vi "sample5(Wrapper).vi"() -> ()   [LabVIEW 2011]
uses:
  <vilib>/Platform/TimedLoop/XDataNode/timing_clust.ctl
  <vilib>/Platform/TimedLoop/XDataNode/nitl_modes.ctl
  <vilib>/Platform/TimedLoop/XDataNode/wakeup.ctl
  <vilib>/Platform/TimedLoop/XDataNode/XDataNode.xnode
  <vilib>/Platform/TimedLoop/XDataNode/XDNodeRunTimeDep.lvlib
panel:
  in  "OffsetTime":u32=20
  out "Present Speed":i16
  in  "waveform":enum16{"sin", "square"}(ring)
  in  "freq":dbl=0.3 format="%_3f"
  in  "Acceleration":u8 max=254
  in  "Goal Speed":i16 min=-1023 max=1023
  out "CycleTime2":dbl format="%.2g"
  out "Load":i16
  in  "TorqueLimit":u16 max=1023
  in  "PID_Gain":u8[](array[numeric])=[0, 0, 0] max=254
  in  "Target ID":u8=1 max=253
  in  "Baudrate":u32=1000000 min=8000 max=3000000
  in  "COM":refnum<visa-resource-name> caption="COMポート"
  out "CycleTime1":dbl format="%.2g"
  out "Current":i16
  in  "wave":bool
  out "CtrlTable":u8[](array[numeric]) format="%02x"
  out "Chart":T1(graph)
  out "STOP2":bool
  out "Present Pos":u16
  in  "STOP":bool
  in  "Goal Pos":u16(knob) scale=0.0..4095.0
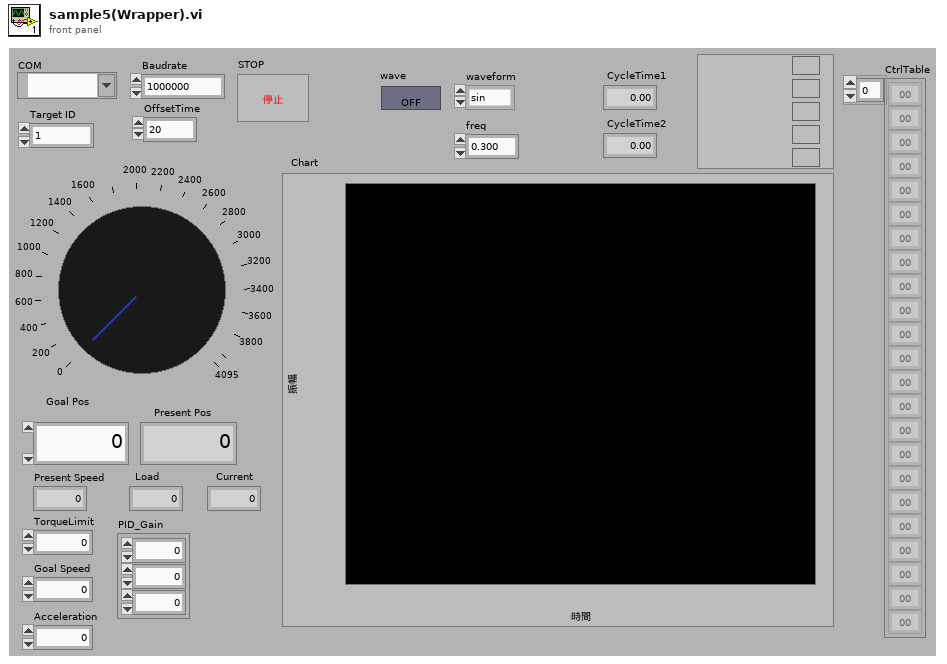
[diagram p1: front panel]
types:
  T1 = cluster{"Goal Pos":u16, "Present Pos":u16, "Current":i16, "Load":i16, "Present Speed":i16}
  T2 = typedef "XDNodeRunTimeDep.lvlib/timing_clust.ctl" = cluster{"Expected End [f-1]":u64, "Actual End [f-1]":u64, "Finished Late? [f-1]":bool, "Expected End [i-1]":u64, "Actual End [i-1]":u64, "Finished Late? [i-1]":bool, "Expected Start [i]":u64, "Actual Start [i]":u64, "Expected Start [f]":u64, "Actual Start [f]":u64, "Source Name":string, "Structure Name":string, "Period":i64, "Deadline":i64, "Offset":i64, "Start":i64, "Priority":i32, "Timeout":i32, "Mode":T3, "Wakeup Reason":T4, "Error":errorcluster, "Source Type":string, "Secondary Source Type":string, "Global End Time":u64, "Global Start Time":u64, "Frame Duration":u64, "Iteration Duration":u64, "Assigned CPU":i32, "I/O Scan Engine Mode":u32}
  T3 = typedef "XDNodeRunTimeDep.lvlib/nitl_modes.ctl" = enum32{"No Change", "Process missed periods, maintain original phase", "Discard missed periods, maintain original phase", "Process missed periods, ignore original phase", "Discard missed periods, ignore original phase"}
  T4 = typedef "XDNodeRunTimeDep.lvlib/wakeup.ctl" = enum32{"Normal", "Aborted", "Asynchronous wakeup", "Timing source error", "Timed loop error", "Timeout"}
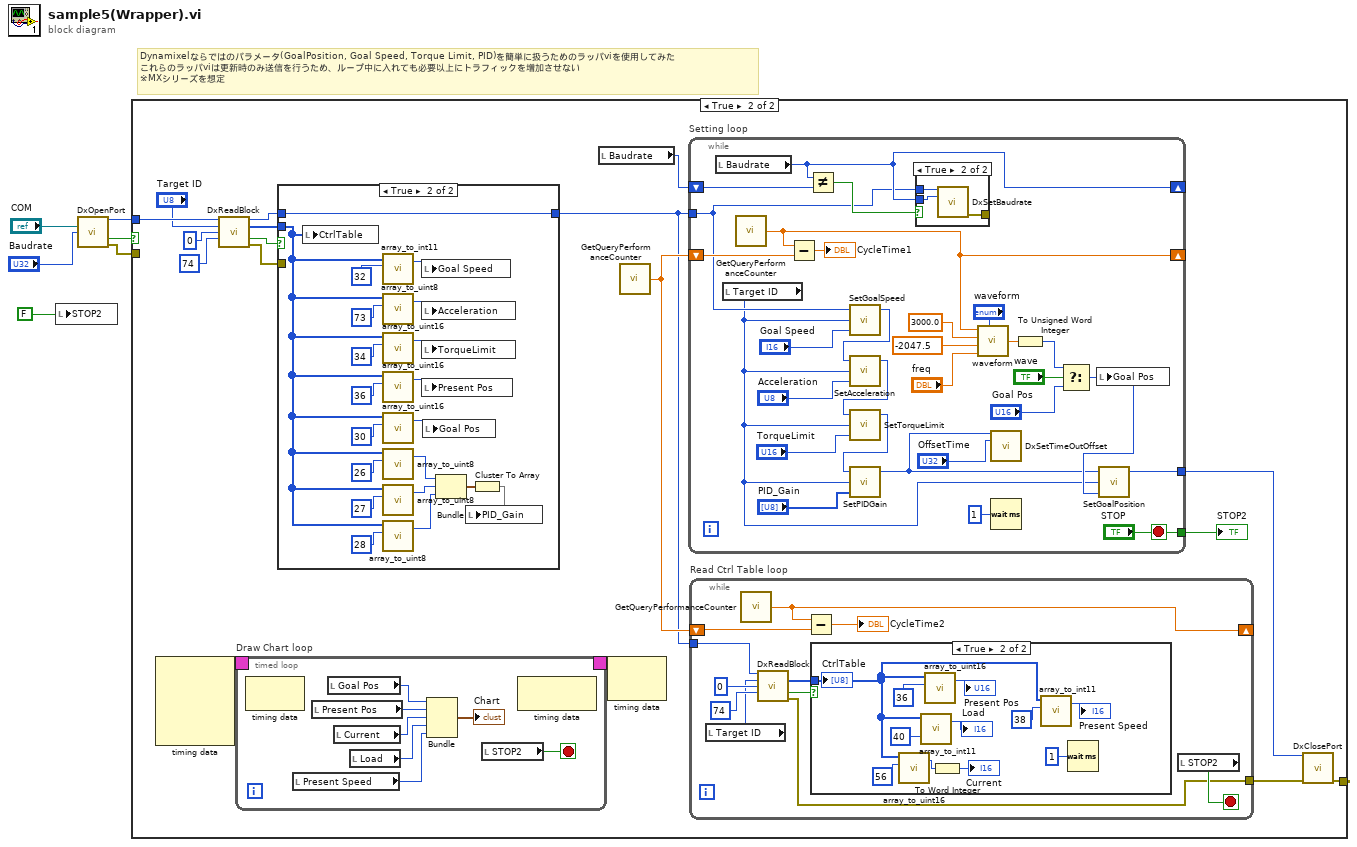
[diagram p0: block diagram]
diagram:
  # "Dynamixelならではのパラメータ(GoalPosition, Goal Speed, Torque Limit, PID)を簡単に扱うためのラッパviを使用してみた\nこれらのラッパviは更新時のみ送信を行うため、ループ中に入れても必要以上にトラフィックを増加させない\n※MXシリーズを想定"
  n1 = local write "STOP2"(FALSE ("停止 3")) -> ()
  n2 = call "DxOpenPort.vi"("port"="COM", "baudrate"="Baudrate") -> ("dvid"=w5:u32, "成功"=w4:bool, "エラー出力"=w6:errorcluster)  [unwired: 11 in]
  n3 = case shown="TRUE" w4 {
    tunnel: w6 -> [_ _]
    tunnel: w5 -> [_ w16]
    tunnel: [_ w9] -> _
    frame False {
    }
    frame True {
      n4 = node-c288() -> (w22:T2)  [unwired: 4 in]
      n5 = call "DxReadBlock.vi"("dvid in"=w16, "id"="Target ID", "address"=u16 0 ("pos"), "size"=u32 74) -> ("dvid out"=w12:u32, "data out"=w14:u8[], "成功"=w13:bool, "エラー出力"=w10:errorcluster)  [unwired: 8 in]
      n6 = timed-loop "Draw Chart loop" {
        timing: w22 -> [_]
        timing-out: [_] -> w21
        stop <- w51 stop-if-true
        n7 = node-c288() -> ()  [unwired: 1 in, 1 out]
        n8 = local read "Present Speed"() -> (w45:i16)
        n9 = local read "Present Pos"() -> (w49:u16)
        n10 = local read "Goal Pos"() -> (w50:u16)
        n11 = local read "Current"() -> (w47:i16)
        n12 = local read "Load"() -> (w46:i16)
        n13 = Bundle("Goal Pos"=w50, "Present Pos"=w49, "Current"=w47, "Load"=w46, "Present Speed"=w45) -> (→"Chart":T1)  [unwired: 1 in]
        n14 = local read "STOP2"() -> (w51:bool)
        n15 = node-c288() -> ()  [unwired: 1 in, 1 out]
      }
      n16 = case shown="TRUE" w13 {
        tunnel: w14 -> [_ w26]
        tunnel: w12 -> [w24 w28]
        tunnel: [w24 w28] -> w11
        tunnel: w10 -> [_ _]
        frame False {
        }
        frame True {
          n17 = local write "CtrlTable"(w26) -> ()
          n18 = call "array_to_int11.vi"("OffsetAddr"=u16 32, "array"=w26) -> ("int16"=w25:i16)  [unwired: 5 in]
          n19 = call "array_to_uint8.vi"("OffsetAddr"=u16 73, "array"=w26) -> ("uint8"=w43:u8)  [unwired: 5 in]
          n20 = call "array_to_uint16.vi"("OffsetAddr"=u16 34, "array"=w26) -> ("uint16"=w37:u16)  [unwired: 5 in]
          n21 = call "array_to_uint16.vi"("OffsetAddr"=u16 36, "array"=w26) -> ("uint16"=w41:u16)  [unwired: 5 in]
          n22 = call "array_to_uint16.vi"("OffsetAddr"=u16 30, "array"=w26) -> ("uint16"=w40:u16)  [unwired: 5 in]
          n23 = call "array_to_uint8.vi"("OffsetAddr"=u16 26, "array"=w26) -> ("uint8"=w33:u8)  [unwired: 5 in]
          n24 = call "array_to_uint8.vi"("OffsetAddr"=u16 27, "array"=w26) -> ("uint8"=w32:u8)  [unwired: 5 in]
          n25 = call "array_to_uint8.vi"("OffsetAddr"=u16 28, "array"=w26) -> ("uint8"=w31:u8)  [unwired: 5 in]
          n26 = local write "Goal Speed"(w25) -> ()
          n27 = local write "Acceleration"(w43) -> ()
          n28 = local write "TorqueLimit"(w37) -> ()
          n29 = local write "Present Pos"(w41) -> ()
          n30 = local write "Goal Pos"(w40) -> ()
          n31 = Bundle("uint8"=w33, "uint8"=w32, "uint8"=w31) -> (w29:cluster{"uint8":u8, "uint8":u8, "uint8":u8})  [unwired: 1 in]
          n32 = Cluster To Array(cluster=w29) -> (array=w30:u8[])
          n33 = local write "PID_Gain"(w30) -> ()
        }
      }
      n34 = local read "Baudrate"() -> (w8:u32)
      n35 = node-c288(w21) -> ()  [unwired: 1 out]
      n36 = call "GetQueryPerformanceCounter.vi"() -> ("performance counter"=w20:dbl)  [unwired: 1 in]
      n37 = while "Setting loop" {
        tunnel: ["STOP"] -> w23
        tunnel: w11 -> [w84]
        shift-right: [w88] -> _
        shift-left: w20 -> [w104]
        tunnel: [w89] -> w19
        shift-right: [w85] -> _
        shift-left: w8 -> [w87]
        stop <- "STOP" stop-if-true
        n38 = local read "Baudrate"() -> (w85:u32)
        n39 = local read "Target ID"() -> (w83:u8)
        n40 = call "GetQueryPerformanceCounter.vi"() -> ("performance counter"=w88:dbl)  [unwired: 1 in]
        n41 = Subtract(x=w88, y=w104) -> (x-y=→"CycleTime1":dbl)
        n42 = Not Equal?(x=w85, y=w87) -> (x != y?=w86:bool)
        n43 = call "SetGoalSpeed.vi"("goal speed"="Goal Speed", "Target ID"=w83, "dvid in"=w84) -> ("dvid out"=w82:u32)  [unwired: 1 in, 1 out]
        n44 = call "SetAcceleration.vi"("acceleration"="Acceleration", "Target ID"=w83, "dvid in"=w82) -> ("dvid out"=w81:u32)  [unwired: 1 in, 1 out]
        n45 = call "SetTorqueLimit.vi"("torque limit"="TorqueLimit", "Target ID"=w83, "dvid in"=w81) -> ("dvid out"=w80:u32)  [unwired: 1 in, 1 out]
        n46 = call "SetPIDGain.vi"("PIDGain"="PID_Gain", "Target ID"=w83, "dvid in"=w80) -> ("dvid out"=w78:u32)  [unwired: 1 in, 1 out]
        n47 = case shown="TRUE" w86 {
          tunnel: w84 -> [_ w109]
          tunnel: w85 -> [_ w108]
          tunnel: [_ w107] -> _
          frame False {
          }
          frame True {
            n48 = call "DxSetBaudrate.vi"("dvid in"=w109, "Baudrate"=w108) -> ("エラー出力"=w107:errorcluster)  [unwired: 11 in, 2 out]
          }
        }
        n49 = call "waveform.vi"("time(ms)"=w88, "amplitude"=3000.0 ("y"), "offset"=-2047.5 ("y"), "frequency"="freq", "waveform"="waveform") -> ("wave"=w95:dbl)
        n50 = call "DxSetTimeOutOffset.vi"("dvid in"=w78, "OffsetTime"="OffsetTime") -> ()  [unwired: 12 in, 2 out]
        n51 = Wait (ms)(milliseconds to wait=u32 1 ("ミリ秒倍数")) -> ()  [unwired: 1 out]
        n52 = To Unsigned Word Integer(number=w95) -> (unsigned 16bit integer=w90:u16)
        n53 = Select(t=w90, s="wave", f="Goal Pos") -> (s? t:f=w96:u16)
        n54 = local write "Goal Pos"(w96) -> ()
        n55 = call "SetGoalPosition.vi"("goal position"=w96, "Target ID"=w83, "dvid in"=w78) -> ("dvid out"=w89:u32)  [unwired: 1 in, 1 out]
      }
      "STOP2" <- w23
      n56 = while "Read Ctrl Table loop" {
        tunnel: w11 -> [w65]
        shift-right: [w57] -> _
        shift-left: w20 -> [w59]
        tunnel: [w56] -> w7
        stop <- w66 stop-if-true
        n57 = local read "Target ID"() -> (w60:u8)
        n58 = call "GetQueryPerformanceCounter.vi"() -> ("performance counter"=w57:dbl)  [unwired: 1 in]
        n59 = call "DxReadBlock.vi"("dvid in"=w65, "id"=w60, "address"=u16 0 ("pos"), "size"=u32 74) -> ("data out"=w62:u8[], "成功"=w61:bool, "エラー出力"=w56:errorcluster)  [unwired: 8 in, 1 out]
        n60 = Subtract(x=w57, y=w59) -> (x-y=→"CycleTime2":dbl)
        n61 = case shown="TRUE" w61 {
          tunnel: w62 -> [_ w68]
          frame False {
          }
          frame True {
            n62 = call "array_to_uint16.vi"("OffsetAddr"=u16 56 ("指標"), "array"=w68) -> ("uint16"=w75:u16)  [unwired: 5 in]
            n63 = call "array_to_int11.vi"("OffsetAddr"=u16 40 ("指標"), "array"=w68) -> ("int16"=→"Load":i16)  [unwired: 5 in]
            n64 = call "array_to_uint16.vi"("OffsetAddr"=u16 36 ("指標"), "array"=w68) -> ("uint16"=→"Present Pos":u16)  [unwired: 5 in]
            n65 = To Word Integer(number=w75) -> (16bit integer=→"Current":i16)
            n66 = call "array_to_int11.vi"("OffsetAddr"=u16 38 ("指標"), "array"=w68) -> ("int16"=→"Present Speed":i16)  [unwired: 5 in]
            n67 = Wait (ms)(milliseconds to wait=u32 1 ("ミリ秒倍数")) -> ()  [unwired: 1 out]
            "CtrlTable" <- w68
          }
        }
        n68 = local read "STOP2"() -> (w66:bool)
      }
      n69 = call "DxClosePort.vi"("dvid"=w19, "エラー入力"=w7) -> ("エラー出力"=w9:errorcluster)  [unwired: 12 in, 1 out]
    }
  }
